vi "Trav_Cluster_to_Row.vi"(4 "Traverse line in":T1 {"Row Duration (mins)" format="%#.1f"; "Row No" min=0; "Trace Gas Concentration (%)" min=0.0 format="%#.2f"; "Emission Rate (l/min)" format="%#.2f"; "Tunnel Speed" format="%#.2f"; "Start X" format="%#.2f"; "Start Y" format="%#.2f"; "Start Z" format="%#.2f"; "End X" format="%#.2f"; "End Y" format="%#.2f"; "End Z" format="%#.2f"; "Averaging time (min)" min=0.0 format="%#.2f"}, 6 "Row Number":i32, 7 "Channel names":string[](array[string])) -> (0 "Traverse line Out":T1 {"Row Duration (mins)" format="%#.1f"; "Row No" min=0; "Trace Gas Concentration (%)" min=0.0 format="%#.2f"; "Emission Rate (l/min)" format="%#.2f"; "Tunnel Speed" format="%#.2f"; "Start X" format="%#.2f"; "Start Y" format="%#.2f"; "Start Z" format="%#.2f"; "End X" format="%#.2f"; "End Y" format="%#.2f"; "End Z" format="%#.2f"; "Averaging time (min)" min=0.0 format="%#.2f"}, 1 "Channel Values Out":string[](array[string]))   [LabVIEW 2012]
uses:
  Traverse_cluster.ctl
  Spacing.ctl
  Controls/Multi_run_mode.ctl
  Globals/Trav_pos_global.vi
  Globals/Meas_global.vi
panel:
  # "X           Y            Z"
  # "Start"
  # "End"
  # "X           Y            Z"
  # "Start"
  # "End"
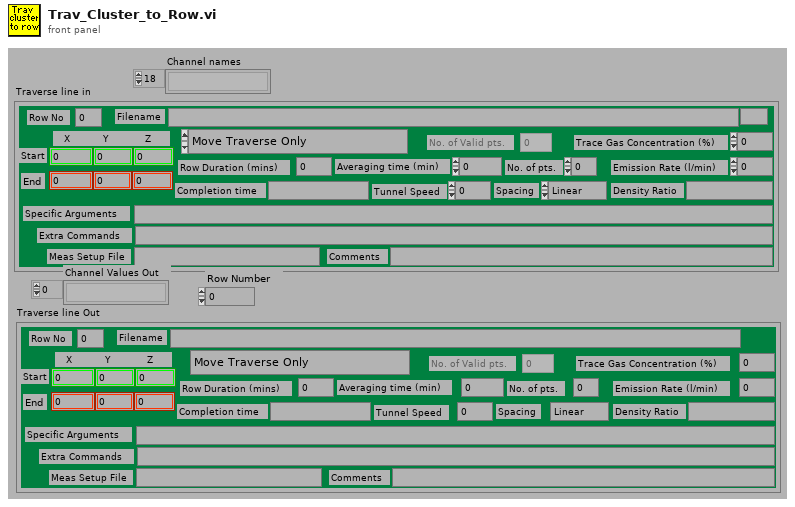
[diagram p1: front panel]
types:
  T1 = typedef "Traverse_cluster.ctl" = cluster{"Start X":dbl, "Start Y":dbl, "Start Z":dbl, "End X":dbl, "End Y":dbl, "End Z":dbl, "No. of pts.":i32, "Spacing":T2, "Filename":path, "Tunnel Speed":dbl, "Averaging time (min)":dbl, "Extra Commands":string, "Specific Arguments":string, "Emission Rate (l/min)":dbl, "Trace Gas Concentration (%)":dbl, "Density Ratio":string, "Comments":string, "Row No":i32, "Row Type Selector":T3, "Completion time":string, "Row Duration (mins)":dbl, "No. of Valid pts.":i32, "Meas Setup File":string}
  T2 = typedef "Spacing.ctl" = enum16{"Linear", "Log", "Gauss", "Specified", "N/A"}
  T3 = typedef "Multi_run_mode.ctl" = enum16{"Move Traverse Only", "Set Tunnel Speed Only", "Set Source Only", "Set Measurement Conditions", "Single Measurement", "Vertical Profile", "Lateral Profile", "Longitudinal Profile", "Explore Volume", "Multi-Axis Profile", "Auto Calibrate", "Meas Fast FID Bkgnd", "Check Beam Power", "Scanning Valve Measurement", "Run VI Named:", "Set ADAM Ch", "Wait (minutes)", "Send Message", "Synchronize With:", "Fall Back to this Row", "Turn Off Row Repeating", "Blank Row", "Traverse 3D Volume"}
  T4 = enum16{"All Channel Names", "Valid Channel Names"}
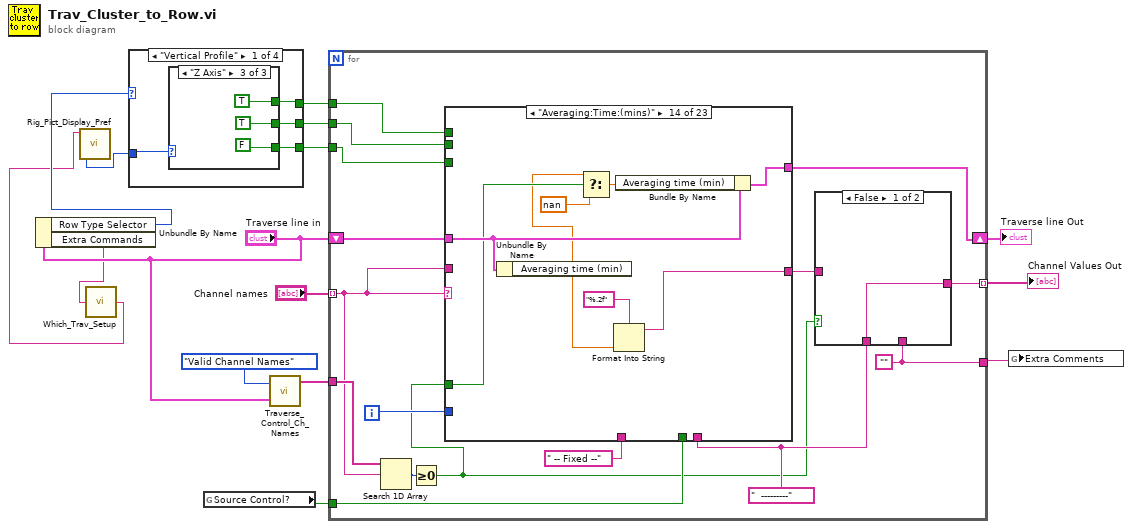
[diagram p0: block diagram]
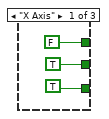
[diagram p2: hidden frame]
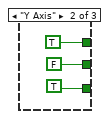
[diagram p3: hidden frame]
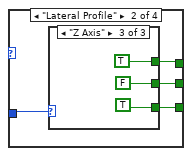
[diagram p4: hidden frame]
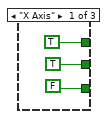
[diagram p5: hidden frame]
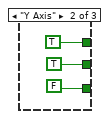
[diagram p6: hidden frame]
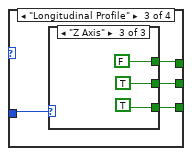
[diagram p7: hidden frame]
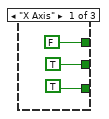
[diagram p8: hidden frame]
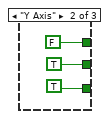
[diagram p9: hidden frame]
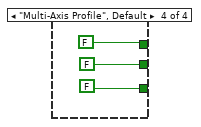
[diagram p10: hidden frame]
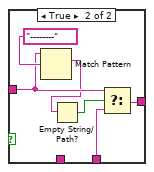
[diagram p11: hidden frame]
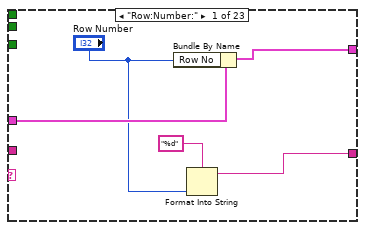
[diagram p12: hidden frame]
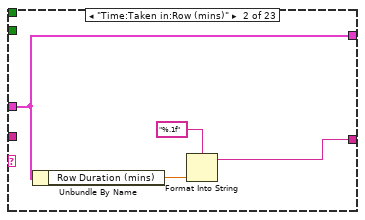
[diagram p13: hidden frame]
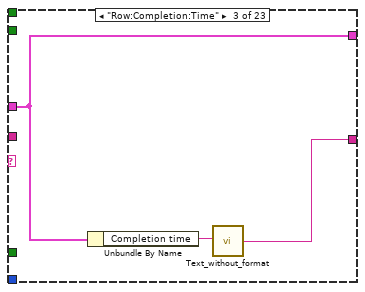
[diagram p14: hidden frame]
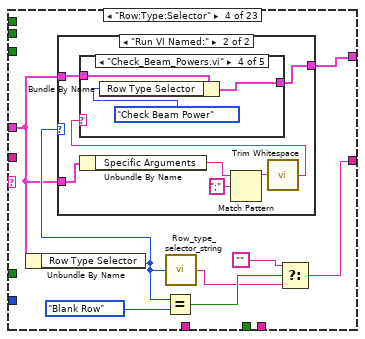
[diagram p15: hidden frame]
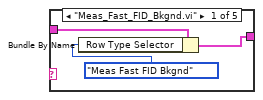
[diagram p17: hidden frame]
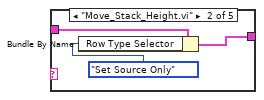
[diagram p18: hidden frame]
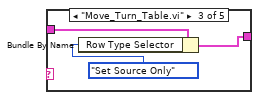
[diagram p19: hidden frame]
diagram:
  n1 = Unbundle By Name("Traverse line in") -> ("Row Type Selector"=w7:T3, "Extra Commands"=w2:string)
  n2 = call "Which_Trav_Setup.vi"("Extra Command String"=w2) -> ("Traverse Setup"=w1:string)
  n3 = call "Rig_Pict_Display_Pref.vi"("Traverse Name"=w1) -> ("Which Axis is vertical?"=w8:enum16{"X Axis", "Y Axis", "Z Axis"})  [unwired: 7 out]
  n4 = case shown="\"Vertical Profile\"" w7 {
    tunnel: [w19 w32 w45 FALSE] -> w6
    tunnel: [w18 w31 w44 FALSE] -> w5
    tunnel: [w17 w30 w43 FALSE] -> w4
    tunnel: w8 -> [w16 w29 w42 _]
    frame "Vertical Profile" {
      n5 = case shown="\"Z Axis\"" w16 {
        tunnel: [FALSE TRUE TRUE] -> w19
        tunnel: [TRUE FALSE TRUE] -> w18
        tunnel: [TRUE TRUE FALSE] -> w17
        frame "X Axis" {
        }
        frame "Y Axis" {
        }
        frame "Z Axis" {
        }
      }
    }
    frame "Lateral Profile" {
      n6 = case shown="\"Z Axis\"" w29 {
        tunnel: [TRUE TRUE TRUE] -> w32
        tunnel: [TRUE TRUE FALSE] -> w31
        tunnel: [FALSE FALSE TRUE] -> w30
        frame "X Axis" {
        }
        frame "Y Axis" {
        }
        frame "Z Axis" {
        }
      }
    }
    frame "Longitudinal Profile" {
      n7 = case shown="\"Z Axis\"" w42 {
        tunnel: [FALSE FALSE FALSE] -> w45
        tunnel: [TRUE TRUE TRUE] -> w44
        tunnel: [TRUE TRUE TRUE] -> w43
        frame "X Axis" {
        }
        frame "Y Axis" {
        }
        frame "Z Axis" {
        }
      }
    }
    frame "Multi-Axis Profile", Default {
    }
  }
  n8 = global read "Trav_pos_global.vi" "Source Control?"() -> (w12:bool)
  n9 = call "Traverse_Control_Ch_Names.vi"("Traverse line"="Traverse line in", "Mode"=T4."Valid Channel Names") -> ("Channel names"=w13:string[])
  n10 = for {
    tunnel: "Channel names" -> [w71] mode=indexing
    tunnel: [w67] -> w15 mode=indexing
    shift-right: [w63] -> w9
    shift-left: "Traverse line in" -> [w73]
    tunnel: w13 -> [w72]
    tunnel: w12 -> [w69]
    tunnel: [w64] -> w10
    tunnel: w6 -> [w61]
    tunnel: w5 -> [w59]
    tunnel: w4 -> [w58]
    i -> [w68]
    w64 = ""
    w65 = "  ---------" ("f")
    n11 = Search 1D Array(1D array=w72, element=w71) -> (index of element=w70:i32)  [unwired: 1 out]
    n12 = Greater Or Equal To 0?(x=w70) -> (x >= 0?=w62:bool)
    n13 = case shown="\"Averaging:Time:(mins)\"" w71 {
      tunnel: w73 -> [w82 w86 w92 w93 w127 w136 w143 w152 w163 w174 w185 w191 w198 w213 w225 w227 w244 w254 w265 w272 w285 w295 w297]
      tunnel: [w84 w88 w90 w97 w126 w134 w142 w150 w159 w169 w180 w193 w199 w215 w219 w228 w236 w251 w262 w269 w278 w288 ""] -> w66
      tunnel: w71 -> [_ _ _ _ _ _ _ _ _ _ _ _ _ _ _ _ _ _ _ _ _ _ w299]
      tunnel: [w83 w86 w92 w94 w128 w135 w144 w151 w162 w173 w184 w192 w196 w214 w224 w234 w243 w255 w266 w275 w286 w296 w297] -> w63
      tunnel: w69 -> [_ _ _ _ _ _ _ _ _ _ _ _ _ _ _ _ _ w253 w263 w274 _ _ _]
      tunnel: w68 -> [_ _ _ _ _ _ _ _ _ _ _ _ _ _ _ _ _ _ _ _ _ _ _]
      tunnel: w65 -> [_ _ _ _ _ _ _ _ _ _ _ _ _ _ w221 w226 w238 w250 w261 w270 w279 w289 _]
      tunnel: w62 -> [_ _ _ _ w124 w132 w138 w147 w157 w167 w178 w189 w195 w211 w222 w230 w239 w248 w259 w271 w281 w291 _]
      tunnel: w61 -> [_ _ _ _ _ _ _ _ w161 _ _ _ _ _ _ _ _ _ _ _ _ _ _]
      tunnel: " -- Fixed --" ("t") -> [_ _ _ _ _ _ _ _ w158 w172 w182 _ _ _ _ _ _ _ _ _ _ _ _]
      tunnel: w59 -> [_ _ _ _ _ _ _ _ _ w171 _ _ _ _ _ _ _ _ _ _ _ _ _]
      tunnel: w58 -> [_ _ _ _ _ _ _ _ _ _ w183 _ _ _ _ _ _ _ _ _ _ _ _]
      frame "Row:Number:" {
        n14 = Bundle By Name(cluster=w82, "Row No"="Row Number") -> (w83:T1)
        n15 = Format Into String(format string="%d", "Row Number") -> (resulting string=w84:string)  [unwired: 2 in, 1 out]
      }
      frame "Time:Taken in:Row (mins)" {
        n16 = Unbundle By Name(w86) -> ("Row Duration (mins)"=w87:dbl)
        n17 = Format Into String(format string="%.1f", w87) -> (resulting string=w88:string)  [unwired: 2 in, 1 out]
      }
      frame "Row:Completion:Time" {
        n18 = Unbundle By Name(w92) -> ("Completion time"=w91:string)
        n19 = call "Text_without_format.vi"("Input string"=w91) -> ("Output string"=w90:string)
      }
      frame "Row:Type:Selector" {
        n20 = Unbundle By Name(w93) -> ("Row Type Selector"=w95:T3)
        n21 = case shown="\"Run VI Named:\"" w95 {
          tunnel: w93 -> [_ w108]
          tunnel: [w101 w107] -> w94
          tunnel: w93 -> [w101 w106]
          frame "Move Traverse Only", Default {
          }
          frame "Run VI Named:" {
            n22 = Unbundle By Name(w108) -> ("Specific Arguments"=w104:string)
            n23 = Match Pattern(string=w104, regular expression=";") -> (before substring=w103:string)  [unwired: 4 out]
            n24 = call <vilib>:"Trim Whitespace.vi"("string"=w103) -> ("trimmed string"=w102:string)  [unwired: 1 in]
            n25 = case shown="\"Check_Beam_Powers.vi\"" w102 {
              tunnel: [w109 w112 w115 w118 w121] -> w107
              tunnel: w106 -> [w111 w113 w116 w119 w121]
              frame "Meas_Fast_FID_Bkgnd.vi" {
                n26 = Bundle By Name(cluster=w111, "Row Type Selector"=Multi_run_mode."Meas Fast FID Bkgnd" ("Mode")) -> (w109:T1)
              }
              frame "Move_Stack_Height.vi" {
                n27 = Bundle By Name(cluster=w113, "Row Type Selector"=Multi_run_mode."Set Source Only" ("Mode")) -> (w112:T1)
              }
              frame "Move_Turn_Table.vi" {
                n28 = Bundle By Name(cluster=w116, "Row Type Selector"=Multi_run_mode."Set Source Only" ("Mode")) -> (w115:T1)
              }
              frame "Check_Beam_Powers.vi" {
                n29 = Bundle By Name(cluster=w119, "Row Type Selector"=Multi_run_mode."Check Beam Power" ("Mode")) -> (w118:T1)
              }
              frame "No Match", Default {
              }
            }
          }
        }
        n30 = Equal?(x=w95, y=Multi_run_mode."Blank Row" ("Mode")) -> (x = y?=w99:bool)
        n31 = call "Row_type_selector_string.vi"("Mode"=w95) -> ("Output string"=w98:string)
        n32 = Select(t="", s=w99, f=w98) -> (s? t:f=w97:string)
      }
      frame "Tunnel:Speed:(m/s)" {
        n33 = Unbundle By Name(w127) -> ("Tunnel Speed"=w123:dbl)
        n34 = Select(t=w123, s=w124, f=nan) -> (s? t:f=w122:dbl)
        n35 = Bundle By Name(cluster=w127, "Tunnel Speed"=w122) -> (w128:T1)
        n36 = Format Into String(format string="%f", w123) -> (resulting string=w126:string)  [unwired: 2 in, 1 out]
      }
      frame "Start at:X:(mm)" {
        n37 = Unbundle By Name(w136) -> ("Start X"=w130:dbl)
        n38 = Select(t=w130, s=w132, f=nan) -> (s? t:f=w131:dbl)
        n39 = Format Into String(format string="%.3f", w130) -> (resulting string=w134:string)  [unwired: 2 in, 1 out]
        n40 = Bundle By Name(cluster=w136, "Start X"=w131) -> (w135:T1)
      }
      frame "Start at:Y:(mm)" {
        n41 = Unbundle By Name(w143) -> ("Start Y"=w139:dbl)
        n42 = Select(t=w139, s=w138, f=nan) -> (s? t:f=w140:dbl)
        n43 = Format Into String(format string="%.3f", w139) -> (resulting string=w142:string)  [unwired: 2 in, 1 out]
        n44 = Bundle By Name(cluster=w143, "Start Y"=w140) -> (w144:T1)
      }
      frame "Start at:Z:(mm)" {
        n45 = Unbundle By Name(w152) -> ("Start Z"=w148:dbl)
        n46 = Select(t=w148, s=w147, f=nan) -> (s? t:f=w146:dbl)
        n47 = Bundle By Name(cluster=w152, "Start Z"=w146) -> (w151:T1)
        n48 = Format Into String(format string="%.3f", w148) -> (resulting string=w150:string)  [unwired: 2 in, 1 out]
      }
      frame "End at:X:(mm)" {
        n49 = Unbundle By Name(w163) -> ("End X"=w154:dbl)
        n50 = Format Into String(format string="%.3f", w154) -> (resulting string=w160:string)  [unwired: 2 in, 1 out]
        n51 = Select(t=w154, s=w157, f=nan) -> (s? t:f=w155:dbl)
        n52 = Bundle By Name(cluster=w163, "End X"=w155) -> (w162:T1)
        n53 = Select(t=w158, s=w161, f=w160) -> (s? t:f=w159:string)
      }
      frame "End at:Y:(mm)" {
        n54 = Unbundle By Name(w174) -> ("End Y"=w166:dbl)
        n55 = Select(t=w166, s=w167, f=nan) -> (s? t:f=w165:dbl)
        n56 = Bundle By Name(cluster=w174, "End Y"=w165) -> (w173:T1)
        n57 = Format Into String(format string="%.3f", w166) -> (resulting string=w170:string)  [unwired: 2 in, 1 out]
        n58 = Select(t=w172, s=w171, f=w170) -> (s? t:f=w169:string)
      }
      frame "End at:Z:(mm)" {
        n59 = Unbundle By Name(w185) -> ("End Z"=w177:dbl)
        n60 = Select(t=w177, s=w178, f=nan) -> (s? t:f=w176:dbl)
        n61 = Bundle By Name(cluster=w185, "End Z"=w176) -> (w184:T1)
        n62 = Format Into String(format string="%.3f", w177) -> (resulting string=w181:string)  [unwired: 2 in, 1 out]
        n63 = Select(t=w182, s=w183, f=w181) -> (s? t:f=w180:string)
      }
      frame "Number:Of:Points" {
        n64 = Unbundle By Name(w191) -> ("No. of pts."=w187:i32)
        n65 = Format Into String(format string="%d", w187) -> (resulting string=w193:string)  [unwired: 2 in, 1 out]
        n66 = Select(t=w187, s=w189, f=0 ("t")) -> (s? t:f=w190:i32)
        n67 = Bundle By Name(cluster=w191, "No. of pts."=w190) -> (w192:T1)
      }
      frame "Point:Spacing:Method" {
        n68 = Unbundle By Name(w198) -> ("Spacing"=w197:T2)
        n69 = case shown="\"N/A\"" w197 {
          tunnel: ["Linear" "Log" "Gauss" "Specified" "N/A"] -> w199
          frame "Linear" {
          }
          frame "Log" {
          }
          frame "Gauss" {
          }
          frame "Specified" {
          }
          frame "N/A" {
          }
        }
        n70 = case shown="True" w195 {
          tunnel: w198 -> [w202 w203]
          tunnel: [w200 w203] -> w196
          frame False {
            n71 = Bundle By Name(cluster=w202, "Spacing"=Spacing."N/A") -> (w200:T1)
          }
          frame True {
          }
        }
      }
      frame "Averaging:Time:(mins)" {
        n72 = Unbundle By Name(w213) -> ("Averaging time (min)"=w209:dbl)
        n73 = Select(t=w209, s=w211, f=nan) -> (s? t:f=w210:dbl)
        n74 = Format Into String(format string="%.2f", w209) -> (resulting string=w215:string)  [unwired: 2 in, 1 out]
        n75 = Bundle By Name(cluster=w213, "Averaging time (min)"=w210) -> (w214:T1)
      }
      frame "Filename:HD:Users" {
        n76 = Unbundle By Name(w225) -> ("Filename"=w223:path)
        n77 = Path To String(path=w223) -> (string=w218:string)
        n78 = call "Text_without_format.vi"("Input string"=w218) -> ("Output string"=w219:string)
        n79 = Select(t=w219, s=w222, f=w221) -> (s? t:f=w220:string)
        n80 = String To Path(string=w220) -> (path=w217:path)
        n81 = Bundle By Name(cluster=w225, "Filename"=w217) -> (w224:T1)
      }
      frame "Specific:Arguments:String" {
        n82 = Unbundle By Name(w227) -> ("Specific Arguments"=w235:string)
        n83 = call "Text_without_format.vi"("Input string"=w235) -> ("Output string"=w231:string)
        n84 = Not Equal?(x=w231, y=w226) -> (x != y?=w233:bool)
        n85 = Select(t=w231, s=w233, f="") -> (s? t:f=w228:string)
        n86 = Select(t=w228, s=w230, f=w226) -> (s? t:f=w229:string)
        n87 = Bundle By Name(cluster=w227, "Specific Arguments"=w229) -> (w234:T1)
      }
      frame "Extra:Commands:String" {
        n88 = Unbundle By Name(w244) -> ("Extra Commands"=w245:string)
        n89 = call "Text_without_format.vi"("Input string"=w245) -> ("Output string"=w240:string)
        n90 = Not Equal?(x=w240, y=w238) -> (x != y?=w242:bool)
        n91 = Select(t=w240, s=w242, f="") -> (s? t:f=w236:string)
        n92 = Select(t=w236, s=w239, f=w238) -> (s? t:f=w237:string)
        n93 = Bundle By Name(cluster=w244, "Extra Commands"=w237) -> (w243:T1)
      }
      frame "Emission:Rate:(l/min)" {
        n94 = Unbundle By Name(w254) -> ("Emission Rate (l/min)"=w247:dbl)
        n95 = Select(t=w247, s=w248, f=nan) -> (s? t:f=w246:dbl)
        n96 = Bundle By Name(cluster=w254, "Emission Rate (l/min)"=w246) -> (w255:T1)
        n97 = Format Into String(format string="%.2f", w247) -> (resulting string=w252:string)  [unwired: 2 in, 1 out]
        n98 = Select(t=w252, s=w253, f=w250) -> (s? t:f=w251:string)
      }
      frame "Trace Gas:Concentration:(%)" {
        n99 = Unbundle By Name(w265) -> ("Trace Gas Concentration (%)"=w258:dbl)
        n100 = Select(t=w258, s=w259, f=nan) -> (s? t:f=w257:dbl)
        n101 = Bundle By Name(cluster=w265, "Trace Gas Concentration (%)"=w257) -> (w266:T1)
        n102 = Format Into String(format string="%.3f", w258) -> (resulting string=w264:string)  [unwired: 2 in, 1 out]
        n103 = Select(t=w264, s=w263, f=w261) -> (s? t:f=w262:string)
      }
      frame "Density:Ratio:" {
        n104 = Unbundle By Name(w272) -> ("Density Ratio"=w276:string)
        n105 = call "Text_without_format.vi"("Input string"=w276) -> ("Output string"=w273:string)
        n106 = Select(t=w273, s=w274, f=w270) -> (s? t:f=w269:string)
        n107 = Select(t=w269, s=w271, f=w270) -> (s? t:f=w268:string)
        n108 = Bundle By Name(cluster=w272, "Density Ratio"=w268) -> (w275:T1)
      }
      frame "Comments::" {
        n109 = Unbundle By Name(w285) -> ("Comments"=w277:string)
        n110 = call "Text_without_format.vi"("Input string"=w277) -> ("Output string"=w282:string)
        n111 = Not Equal?(x=w282, y=w279) -> (x != y?=w284:bool)
        n112 = Select(t=w282, s=w284, f="") -> (s? t:f=w278:string)
        n113 = Select(t=w278, s=w281, f=w279) -> (s? t:f=w280:string)
        n114 = Bundle By Name(cluster=w285, "Comments"=w280) -> (w286:T1)
      }
      frame "Measurement:Setup:File" {
        n115 = Unbundle By Name(w295) -> ("Meas Setup File"=w287:string)
        n116 = call "Text_without_format.vi"("Input string"=w287) -> ("Output string"=w292:string)
        n117 = Not Equal?(x=w292, y=w289) -> (x != y?=w294:bool)
        n118 = Select(t=w292, s=w294, f="") -> (s? t:f=w288:string)
        n119 = Select(t=w288, s=w291, f=w289) -> (s? t:f=w290:string)
        n120 = Bundle By Name(cluster=w295, "Meas Setup File"=w290) -> (w296:T1)
      }
      frame "No match", Default {
        n121 = call "Was_string_matched.vi"("Variable name"=w299) -> ()  [unwired: 2 in]
      }
    }
    n122 = case shown="False" w62 {
      tunnel: [w74 w79] -> w67
      tunnel: w66 -> [_ w77]
      tunnel: w65 -> [w74 _]
      tunnel: w64 -> [_ w80]
      frame False {
      }
      frame True {
        n123 = Match Pattern(string=w77, regular expression="--------" ("f")) -> (match substring=w76:string)  [unwired: 4 out]
        n124 = Empty String/Path?(string/path=w76) -> (empty?=w75:bool)
        n125 = Select(t=w77, s=w75, f=w80) -> (s? t:f=w79:string)
      }
    }
  }
  "Channel Values Out" <- w15
  "Traverse line Out" <- w9
  n126 = global write "Meas_global.vi" "Extra Comments"(w10) -> ()
